vi "Error Message.vi"(8 "error in (no error)":errorcluster, 10 "error code":i32, 11 "Connection in":refnum<class "Connection.lvclass">) -> (0 "error out":errorcluster, 3 "Connection out":refnum<class "Connection.lvclass">)   [LabVIEW 2011, in "SQLite.lvlib" / "Connection.lvclass"]
uses:
  Connection.lvclass
  Connection.lvclass/Connection.ctl
  SQLite.lvlib
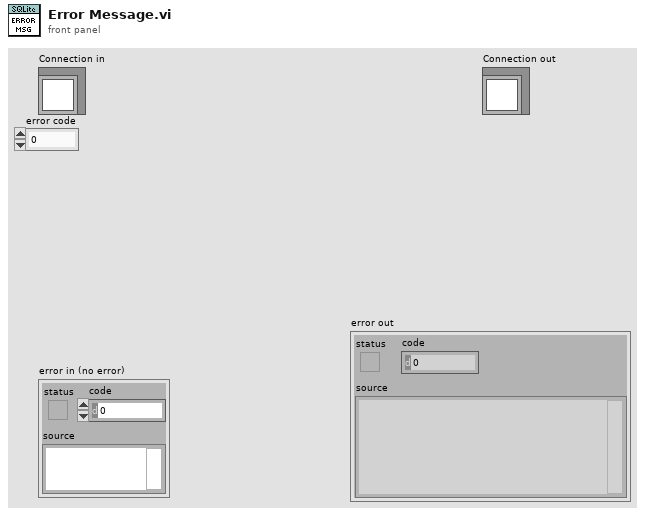
[diagram p1: front panel]
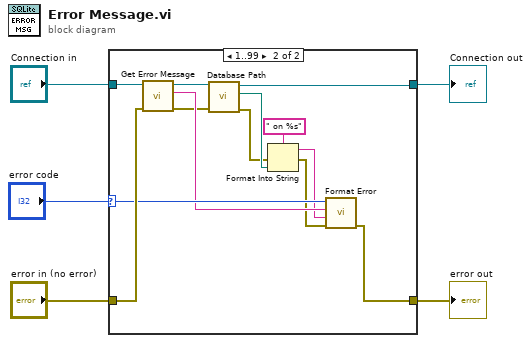
[diagram p0: block diagram]
diagram:
  n1 = case shown="1..99" "error code" {
    selector: "error code" -> [_ w18]
    tunnel: "Connection in" -> [w6 w20]
    tunnel: "error in (no error)" -> [w7 w19]
    tunnel: [w7 w16] -> w2
    tunnel: [w6 w13] -> w1
    frame 0, Default {
    }
    frame 1..99 {
      n2 = call "Get Error Message.vi"("error in (no error)"=w19, "Connection in"=w20) -> ("error out"=w14:errorcluster, "error message"=w17:string, "Connection out"=w15:refnum<class "Connection.lvclass">)  [unwired: 7 in]
      n3 = call "Database Path.vi"("error in (no error)"=w14, "Connection in"=w15) -> ("error out"=w9:errorcluster, "Path to Database"=w12:path, "Connection out"=w13:refnum<class "Connection.lvclass">)  [unwired: 7 in]
      n4 = Format Into String(format string=" on %s", error in=w9, w12) -> (resulting string=w10:string, error out=w8:errorcluster)  [unwired: 1 in]
      n5 = call "Format Error.vi"("error in (no error)"=w8, "Additional source description"=w10, "error message"=w17, "error code"=w18) -> ("error out"=w16:errorcluster)  [unwired: 7 in]
    }
  }
  "error out" <- w2
  "Connection out" <- w1
